vi "Set Buffer Filling Mode.vi"(0 "VISA resource name":refnum<visa-resource-name>, 5 "Buffer Name (defbuffer1)":string="defbuffer1", 7 "Fill Type":u16(ring) items=["Continuous", "Once"], 11 "error in (no error)":errorcluster) -> (4 "VISA resource name out":refnum<visa-resource-name>, 15 "error out":errorcluster)   [LabVIEW 2017, in "Keithley 2450.lvlib"]
doc: "This Vi determines if a reading buffer is filled continuously or is filled once and stops."
uses:
  Keithley 2450.lvlib
panel:
  out "Status":sgl[](array[numeric])
  out "Timestamp":sgl[](array[numeric])
  out "Resistance":sgl[](array[numeric])
  out "Current":sgl[](array[numeric])
  out "Voltage":sgl[](array[numeric])
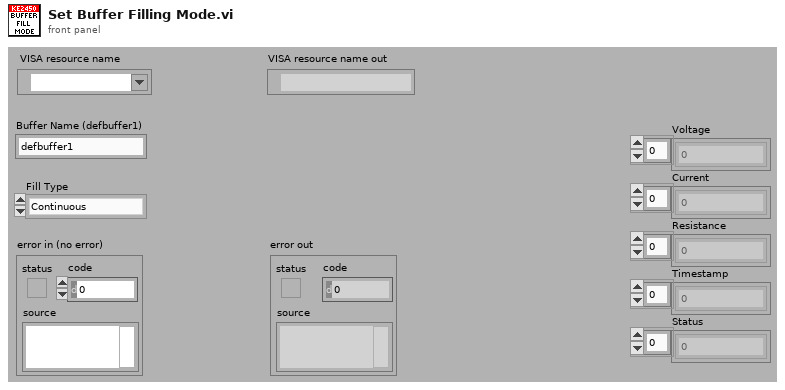
[diagram p1: front panel]
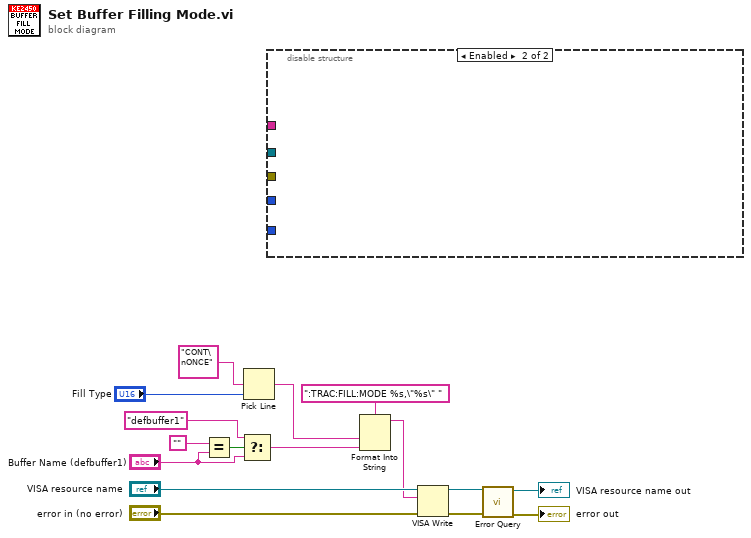
[diagram p0: block diagram]
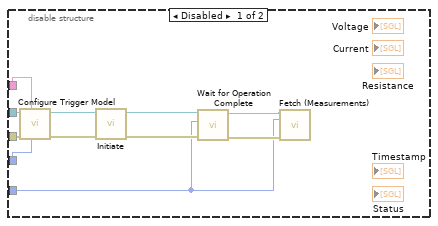
[diagram p2: hidden frame]
diagram:
  n1 = Equal?(x="", y="Buffer Name (defbuffer1)") -> (x = y?=w13:bool)
  n2 = Select(t="defbuffer1", s=w13, f="Buffer Name (defbuffer1)") -> (s? t:f=w1:string)
  n3 = Pick Line(multi-line string="CONT\nONCE", line index="Fill Type") -> (output string=w3:string)  [unwired: 1 in]
  n4 = disable-structure shown="Enabled" {
    disable-tunnel: _ -> [w23 _]
    disable-tunnel: _ -> [w22 _]
    disable-tunnel: _ -> [w21 _]
    disable-tunnel: _ -> [w20 _]
    disable-tunnel: _ -> [w17 _]
    frame Disabled {
      n5 = call "Configure Trigger Model.vi"("Trigger Count (1)"=w22, "Buffer Name (defbuffer1)"=w17, "error in (no error)"=w20, "VISA resource name"=w21) -> ("error out"=w18:errorcluster, "VISA resource name out"=w19:refnum<visa-resource-name>)  [unwired: 6 in]
      n6 = call "Initiate.vi"("error in (no error)"=w18, "VISA resource name"=w19) -> ("error out"=w26:errorcluster, "VISA resource name out"=w27:refnum<visa-resource-name>)  [unwired: 8 out]
      n7 = call "Wait for Operation Complete.vi"("error in (no error)"=w26, "Timeout (10000 ms)"=w23, "VISA resource name"=w27) -> ("error out"=w25:errorcluster, "VISA resource name out"=w24:refnum<visa-resource-name>)  [unwired: 7 out]
      n8 = call "Fetch (Measurements).vi"("VISA resource name"=w24, "Timeout (10000 ms)"=w23, "error in (no error)"=w25) -> ()  [unwired: 2 in, 11 out]
    }
    frame Enabled {
    }
  }
  n9 = Format Into String(format string=":TRAC:FILL:MODE %s,\"%s\" " ("Fetch Measurement"), w3, w1) -> (resulting string=w2:string)  [unwired: 2 in, 1 out]
  n10 = VISA Write(VISA resource name="VISA resource name", write buffer=w2, error in (no error)="error in (no error)") -> (VISA resource name out=w8:refnum<visa-resource-name>, error out=w7:errorcluster)  [unwired: 1 out]
  n11 = call "Error Query.vi"("error in (no error)"=w7, "VISA resource name"=w8) -> ("error out"=→"error out":errorcluster, "VISA resource name out"=→"VISA resource name out":refnum<visa-resource-name>)  [unwired: 8 out]
